vi "Configure Parameter MARK.vi"(7 "PARAM":enum16{"WAVE", "HIGH"}(ring), 8 "error in (no error)":errorcluster, 9 "STAT@HIGH":enum16{"ON", "OFF"}(ring), 10 "STAT@WAVE":enum16{"SQU", "PULS", "TRI", "LINE"}(ring), 11 "VISA resource name":refnum<visa-resource-name>) -> (0 "error out":errorcluster, 3 "VISA resource name out":refnum<visa-resource-name>)   [LabVIEW 2018, in "Fluke 9500B.lvlib"]
uses:
  <instrlib>/Fluke 9500B/Fluke 9500B.lvlib
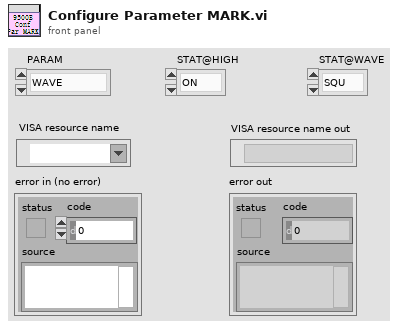
[diagram p1: front panel]
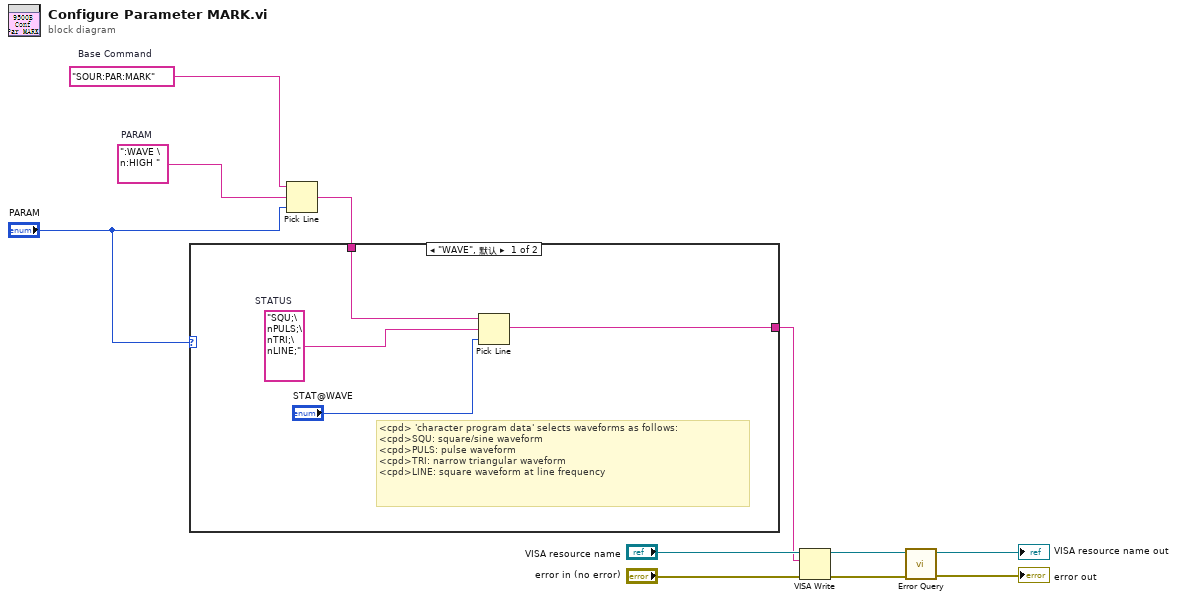
[diagram p0: block diagram]
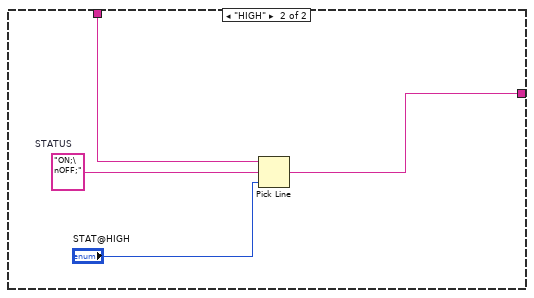
[diagram p2: hidden frame]
diagram:
  w8 = ":WAVE \n:HIGH "  # PARAM
  w9 = "SOUR:PAR:MARK"  # Base Command
  n1 = Pick Line(string ("")=w9, multi-line string=w8, line index="PARAM") -> (output string=w7:string)
  n2 = case shown="\"WAVE\", 默认" "PARAM" {
    tunnel: w7 -> [w13 w17]
    tunnel: [w12 w16] -> w6
    frame "WAVE", Default {
      w15 = "SQU;\nPULS;\nTRI;\nLINE;"  # STATUS
      # "<cpd> 'character program data' selects waveforms as follows: \n<cpd>SQU: square/sine waveform \n<cpd>PULS: pulse waveform \n<cpd>TRI: narrow triangular waveform \n<cpd>LINE: square waveform at line frequency"
      n3 = Pick Line(string ("")=w13, multi-line string=w15, line index="STAT@WAVE") -> (output string=w12:string)
    }
    frame "HIGH" {
      w18 = "ON;\nOFF;"  # STATUS
      n4 = Pick Line(string ("")=w17, multi-line string=w18, line index="STAT@HIGH") -> (output string=w16:string)
    }
  }
  n5 = VISA Write(VISA resource name="VISA resource name", write buffer=w6, error in (no error)="error in (no error)") -> (VISA resource name out=w4:refnum<visa-resource-name>, error out=w3:errorcluster)  [unwired: 1 out]
  n6 = call <instrlib>:"Error Query.vi"("error in (no error)"=w3, "VISA resource name"=w4) -> ("error out"=→"error out":errorcluster, "VISA resource name out"=→"VISA resource name out":refnum<visa-resource-name>)  [unwired: 6 in, 2 out]
